vi "Send command Get Pin.vi"(7 "Marca":string, 8 "error in (no error)":errorcluster, 9 "Pin":string, 10 "Puerto":string, 11 "Serial Device in":refnum<class "Serial Device.lvclass">) -> (0 "error out":errorcluster, 1 "Command":string, 2 "Expected response":string, 3 "Serial Device out":refnum<class "Serial Device.lvclass">)   [LabVIEW 2020, in "Serial Device.lvclass"]
doc: "Se tiene dentro el comando para obtener el estatus del pin y este sera solo para mandarlo a llamar"
uses:
  Serial Device.lvclass
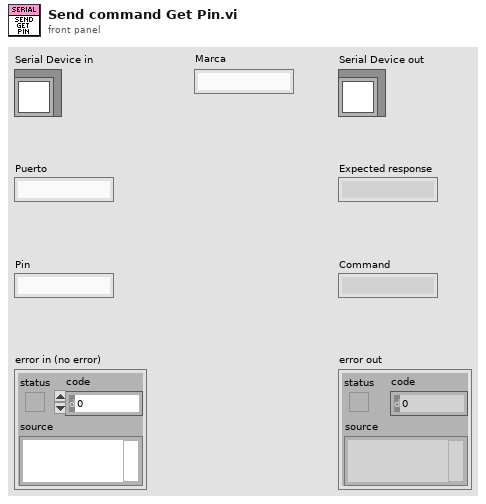
[diagram p1: front panel]
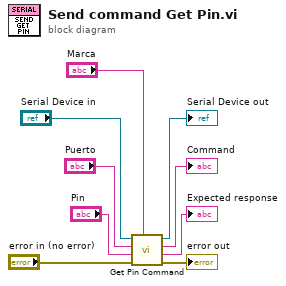
[diagram p0: block diagram]
diagram:
  n1 = call "Get Pin Command.vi"("Marca"="Marca", "error in (no error)"="error in (no error)", "Pin"="Pin", "Puerto"="Puerto", "Serial Device in"="Serial Device in") -> ("error out"=→"error out":errorcluster, "Expected response"=→"Expected response":string, "Command"=→"Command":string, "Serial Device out"=→"Serial Device out":refnum<class "Serial Device.lvclass">)  [unwired: 3 in]
